vi "PicoScope4000GetValuesOverlapped.vi"(5 "Segment Range":T1 {"toSegmentIndex" format="%.4p"; "fromSegmentIndex" format="%.4p"}, 7 "Buffer and Transfer Settings":T2 {"Down-Sample Mode" items=["RAW none", "None", "Aggregate", "Decimate", "Average"]; "Down Sample Ratio" step=1; "Samples" format="%_6p"}, 8 "error in (no error)":errorcluster, 11 "handle in":i16) -> (0 "error out":errorcluster, 3 "handle out":i16, 4 "overflow":i16 format="%010b", 6 "noOfSamples":u64)   [LabVIEW 2009]
doc: "Calls GetValuesOverlapped"
uses:
  ps4000a.dll
  shared/Buffer and Transfer Settings.ctl
  shared/Segment Range.ctl
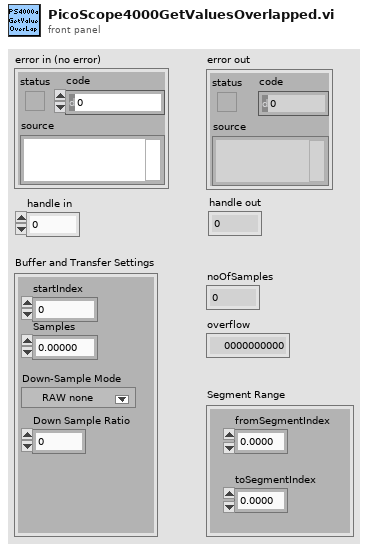
[diagram p1: front panel]
types:
  T1 = typedef "Segment Range.ctl" = cluster{"fromSegmentIndex":u64, "toSegmentIndex":u64}
  T2 = typedef "Buffer and Transfer Settings.ctl" = cluster{"startIndex":u64, "Samples":u64, "Down Sample Ratio":u64, "Down-Sample Mode":u32}
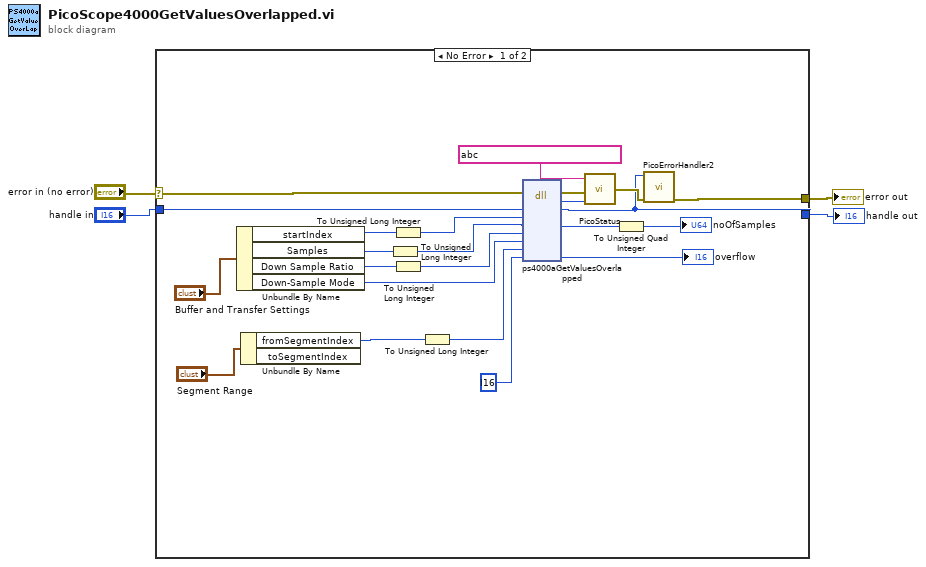
[diagram p0: block diagram]
diagram:
  n1 = case shown="No Error" "error in (no error)" {
    selector: "error in (no error)" -> [w22 w28]
    tunnel: "handle in" -> [w21 w29]
    tunnel: [w7 w29] -> w4
    tunnel: [w20 w28] -> w3
    frame #0 {
      n2 = Unbundle By Name("Buffer and Transfer Settings") -> ("startIndex"=w15:u64, "Samples"=w13:u64, "Down Sample Ratio"=w14:u64, "Down-Sample Mode"=w9:u32)
      n3 = Unbundle By Name("Segment Range") -> ("fromSegmentIndex"=w17:u64)  [unwired: 1 out]
      n4 = To Unsigned Long Integer(number=w13) -> (unsigned 32bit integer=w11:u32)
      n5 = To Unsigned Long Integer(number=w15) -> (unsigned 32bit integer=w12:u32)
      n6 = To Unsigned Long Integer(number=w14) -> (unsigned 32bit integer=w10:u32)
      n7 = To Unsigned Long Integer(number=w17) -> (unsigned 32bit integer=w16:u32)
      n8 = dll-call lib="ps4000a.dll" fn="ps4000aGetValuesOverlapped" ("ps3000.dll:_ps3000_open_unit@0")(error in=w22, "handle"=w21, "startIndex"=w12, "noOfSamples"=w11, "downSampleRatio"=w10, "downSampleRatioMode"=w9, "segmentIndex"=w16, "overflow"=i16 ?) -> (error out=w26:errorcluster, "PICO_STATUS"=w8:u32, "handle"=w7:i16, "noOfSamples"=w6:u32, "overflow"=→"overflow":i16)  [unwired: 6 in, 1 out]
      n9 = call "PicoStatus.vi"("PICO STATUS"=w8, "error in"=w26, "source"=string ?) -> ("error out"=w27:errorcluster)
      n10 = To Unsigned Quad Integer(1:w6) -> (0:→"noOfSamples":u64)
      n11 = call "PicoErrorHandler2.vi"("error in (no error)"=w27, "handle In"=w7) -> ("error out"=w20:errorcluster)  [unwired: 9 in]
    }
    frame #1 {
    }
  }
  "error out" <- w3
  "handle out" <- w4
